vi "Drive Precision Filter.vi"(9 "Precision Button":bool, 10 "Y Axis":dbl, 11 "X Axis":dbl) -> (2 "Y Axis Output":dbl, 3 "X Axis Output":dbl)   [LabVIEW 2014]
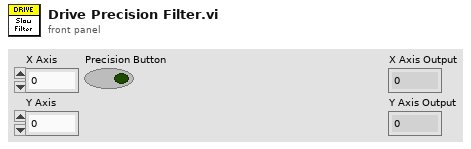
[diagram p1: front panel]
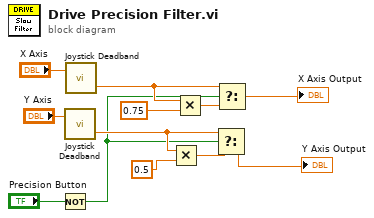
[diagram p0: block diagram]
diagram:
  n1 = Not(x="Precision Button") -> (.not. x?=w1:bool)
  n2 = call "Joystick Deadband.vi"("Joystick Value"="Y Axis") -> ("Joystick Output"=w4:dbl)  [unwired: 1 in]
  n3 = call "Joystick Deadband.vi"("Joystick Value"="X Axis") -> ("Joystick Output"=w6:dbl)  [unwired: 1 in]
  n4 = Multiply(x=w4, y=0.5) -> (x*y=w11:dbl)
  n5 = Multiply(x=w6, y=0.75) -> (x*y=w12:dbl)
  n6 = Select(t=w4, s=w1, f=w11) -> (s? t:f=→"Y Axis Output":dbl)
  n7 = Select(t=w6, s=w1, f=w12) -> (s? t:f=→"X Axis Output":dbl)
